vi "Spawn Child placeholder.vi"(7 "Actor in":refnum<class "Actor.lvclass">) -> (0 "Error out":errorcluster, 5 "Actor out":refnum<class "Actor.lvclass">)   [LabVIEW 2025, in "_Template.lvlib" / "Templates.lvlib" / "TEMPLATE Actor.lvlib"]
uses:
  TEMPLATE Actor.lvlib
  jettl/jettl/Actor/Actor.lvclass
  Static Child UIDs.ctl
  jettl/jettl/jettl.lvlib
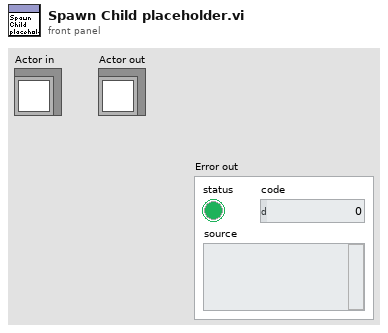
[diagram p1: front panel]
types:
  T1 = typedef "_Template.lvlib/Templates.lvlib/TEMPLATE Actor.lvlib/Static Child UIDs.ctl" = enum16{"placeholder"}
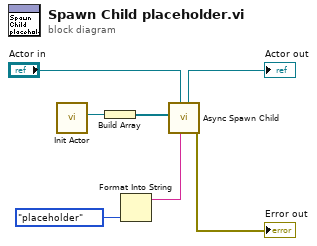
[diagram p0: block diagram]
diagram:
  n1 = call "Init Actor.vi"() -> ("Actor"=w5:refnum<class "Actor.lvclass">)  [unwired: 11 in]
  n2 = Build Array(w5) -> (w4:refnum<class "Actor.lvclass">[])
  n3 = Format Into String(Static_Child_UIDs."placeholder" ("Static Child UIDs")) -> (resulting string=w3:string)  [unwired: 3 in, 1 out]
  n4 = call "Async Spawn Child.vi"("UID"=w3, "Actor in"="Actor in", "Local Layers"=w4) -> ("Error out"=→"Error out":errorcluster, "Actor out"=→"Actor out":refnum<class "Actor.lvclass">)  [unwired: 7 in]
